vi "Initialize.vi"(5 "enableDefaultFile":bool, 6 "hostApplicationPath":path, 7 "configFilePath":path, 8 "error in (no error)":errorcluster, 9 "defaultFileAppender":T2={"common"={"id"="", "threshold"=enum."INFO", "filter"={"mode"=enum."Mirror", "levelMin"=enum."INFO", "levelMax"=enum."INFO", "tagPrefix"=""}, "queueBound"=-1, "dropPolicy"=enum."DropOldest", "useUTC"=FALSE}, "file"={"rootFolder"=path "", "maxFileSize"=-1, "maxFileCount"=-1, "baseName"="", "extension"="", "delimiter"="", "calendarFolderTree"=FALSE}}, 10 "initialGlobalThreshold":T1=enum."INFO", 11 "Logger in":refnum<class "Logger.lvclass">) -> (0 "error out":errorcluster, 3 "Logger out":refnum<class "Logger.lvclass">)   [LabVIEW 2026, in "Lumberjack.lvlib" / "Logger.lvclass"]
doc: "Launches the logging system and returns a ready logger.\nBundles the launch inputs (initial global threshold, host application path, optional config file, notifiers) into ManagerLaunchInputs, launches the LogManager as a root actor (SetLaunchInputs + Launch Root Actor), stores the instance as the process default (SetProcessDefault), and blocks on WaitForSnapshot(AnySnapshot) until the manager publishes its first Snapshot so the next Log reaches a live tree; starts the default file appender when enableDefaultFile is TRUE.\nLumberjack.lvlib, Logger.lvclass, public."
uses:
  Logger.lvclass
  TypeDefs/FileAppenderConfig.ctl
  TypeDefs/AppenderConfig.ctl
  TypeDefs/Severity.ctl
  TypeDefs/Filter.ctl
  TypeDefs/FilterMode.ctl
  TypeDefs/DropPolicy.ctl
  TypeDefs/FileConfig.ctl
  Core/LogManager/LogManager.lvclass/LogManager.lvclass
  C:/Program Files/National Instruments/LabVIEW 2026/vi.lib/ActorFramework/Actor/Actor.lvclass
  TypeDefs/Snapshot.ctl
  <vilib>/ActorFramework/Message Enqueuer/Message Enqueuer.lvclass
  TypeDefs/SnapshotWaitMode.ctl
  TypeDefs/ManagerLaunchInputs.ctl
  Logger.lvclass/Logger.ctl
  <vilib>/ActorFramework/Actor/Actor.lvclass
  Lumberjack.lvlib
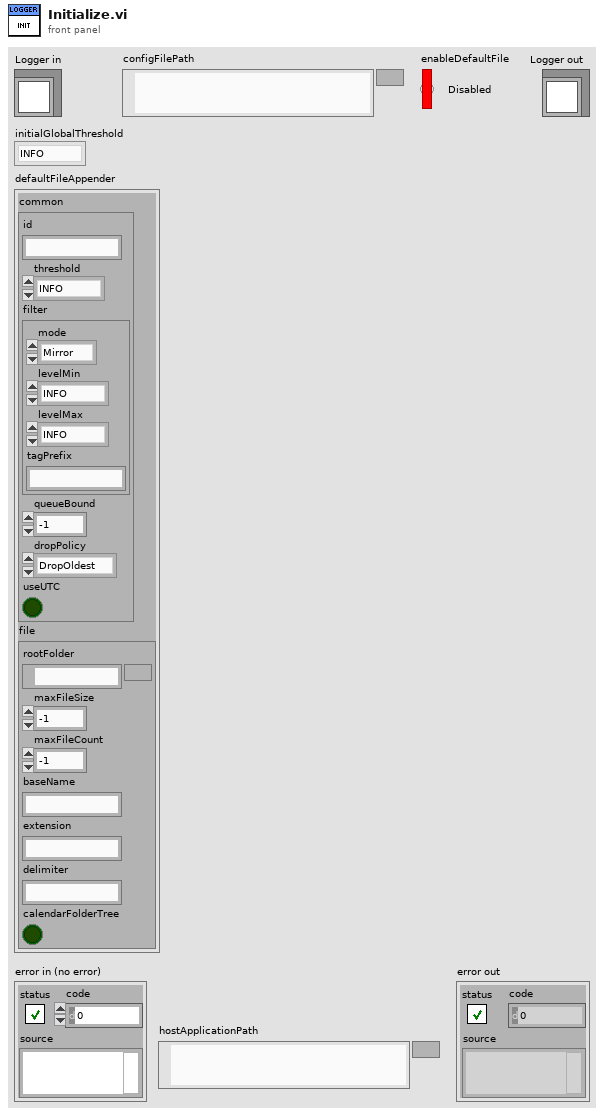
[diagram p1: front panel]
types:
  T1 = typedef "Lumberjack.lvlib/Severity.ctl" = enum16{"OFF", "FATAL", "ERROR", "WARN", "INFO", "DEBUG", "TRACE", "ALL"}
  T2 = typedef "Lumberjack.lvlib/FileAppenderConfig.ctl" = cluster{"common":T3, "file":T7}
  T3 = typedef "Lumberjack.lvlib/AppenderConfig.ctl" = cluster{"id":string, "threshold":T1, "filter":T4, "queueBound":i32, "dropPolicy":T6, "useUTC":bool}
  T4 = typedef "Lumberjack.lvlib/Filter.ctl" = cluster{"mode":T5, "levelMin":T1, "levelMax":T1, "tagPrefix":string}
  T5 = typedef "Lumberjack.lvlib/FilterMode.ctl" = enum16{"Mirror", "Routed"}
  T6 = typedef "Lumberjack.lvlib/DropPolicy.ctl" = enum16{"DropOldest", "DropNewest", "LevelAware"}
  T7 = typedef "Lumberjack.lvlib/FileConfig.ctl" = cluster{"rootFolder":path, "maxFileSize":i64, "maxFileCount":i32, "baseName":string, "extension":string, "delimiter":string, "calendarFolderTree":bool}
  T8 = typedef "Lumberjack.lvlib/SnapshotWaitMode.ctl" = enum16{"AnySnapshot", "IDPresent", "IDAbsent"}
  T9 = typedef "Lumberjack.lvlib/ManagerLaunchInputs.ctl" = cluster{"initialGlobalThreshold":T1, "hostApplicationPath":path, "configFilePath":path, "snapshotNotifier":refnum<notifier>, "stoppedNotifier":refnum<notifier>}
  T10 = typedef "Lumberjack.lvlib/Snapshot.ctl" = cluster{"globalThreshold":T1, "appenders":cluster{"id":string, "enqueuer":refnum<class "Message Enqueuer.lvclass">}[]}
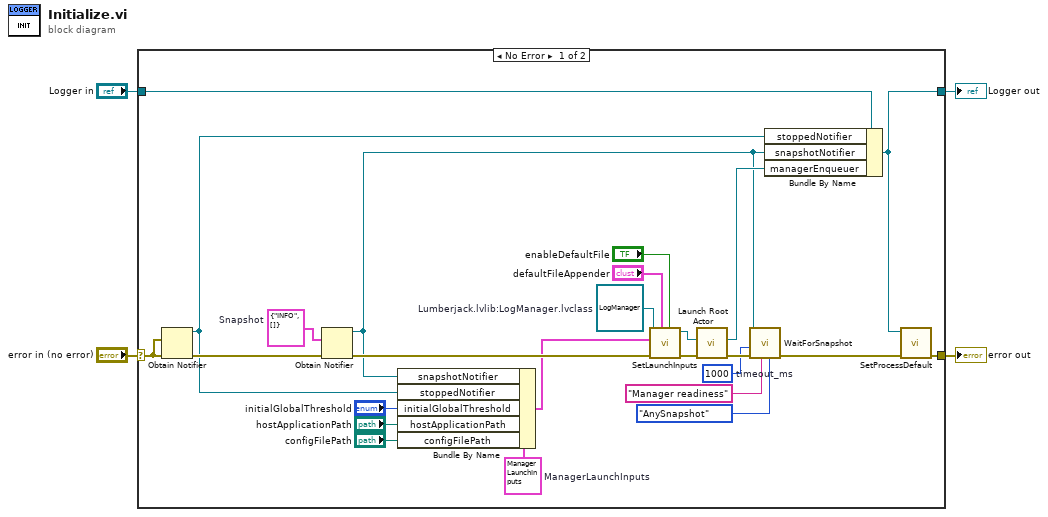
[diagram p0: block diagram]
diagram:
  n1 = case shown="No Error" "error in (no error)" {
    selector: "error in (no error)" -> [w15 w31]
    tunnel: [w24 w31] -> w3
    tunnel: [w23 w30] -> w1
    tunnel: "Logger in" -> [w25 w30]
    frame No Error {
      w8 = T9 {"initialGlobalThreshold"=enum."INFO", "hostApplicationPath"=path "", "configFilePath"=path "", "snapshotNotifier"=refnum, "stoppedNotifier"=refnum}  # ManagerLaunchInputs
      w18 = 1000  # timeout_ms
      w27 = T10 {"globalThreshold"=enum."INFO", "appenders"=[]}  # Snapshot
      w29 = refnum<class "LogManager.lvclass"> refnum  # Lumberjack.lvlib:LogManager.lvclass
      n2 = Obtain Notifier(notification data type=w15, error in (no error)=w15) -> (notifier out=w6:refnum<notifier>, error out=w16:errorcluster)  [unwired: 2 in, 1 out]
      n3 = Obtain Notifier(notification data type=w27, error in (no error)=w16) -> (notifier out=w7:refnum<notifier>, error out=w26:errorcluster)  [unwired: 2 in, 1 out]
      n4 = Bundle By Name(cluster=w8, "snapshotNotifier"=w7, "stoppedNotifier"=w6, "initialGlobalThreshold"="initialGlobalThreshold", "hostApplicationPath"="hostApplicationPath", "configFilePath"="configFilePath") -> (w5:T9)
      n5 = call "SetLaunchInputs.vi"("enableDefaultFile"="enableDefaultFile", "defaultFileAppender"="defaultFileAppender", "error in (no error)"=w26, "ManagerLaunchInputs"=w5, "LogManager in"=w29) -> ("error out"=w28:errorcluster, "LogManager out"=w12:refnum<class "LogManager.lvclass">)  [unwired: 5 in]
      n6 = call <vilib>:"Launch Root Actor.vi"("error in (no error)"=w28, "Actor"=w12) -> ("error out"=w21:errorcluster, "Actor's Enqueuer"=w22:refnum<class "Message Enqueuer.lvclass">)  [unwired: 8 in]
      n7 = call "WaitForSnapshot.vi"("snapshotWaitMode"=SnapshotWaitMode."AnySnapshot" ("SnapshotWaitMode"), "context"="Manager readiness" ("Context"), "error in (no error)"=w21, "timeout_ms"=w18, "snapshotNotifier"=w7) -> ("error out"=w20:errorcluster)  [unwired: 5 in, 1 out]
      n8 = Bundle By Name(cluster=w25, "stoppedNotifier"=w6, "snapshotNotifier"=w7, "managerEnqueuer"=w22) -> (w23:refnum<class "Logger.lvclass">)
      n9 = call "SetProcessDefault.vi"("error in (no error)"=w20, "Logger in"=w23) -> ("error out"=w24:errorcluster)  [unwired: 9 in]
    }
    frame Error {
    }
  }
  "error out" <- w3
  "Logger out" <- w1
